vi "CreateObstacleMap.vi"(8 "Base Map":dbl[][](array[numeric]), 11 "Obstacles":T1) -> (3 "Obstacle Map":dbl[][](array[numeric]))   [LabVIEW 2011]
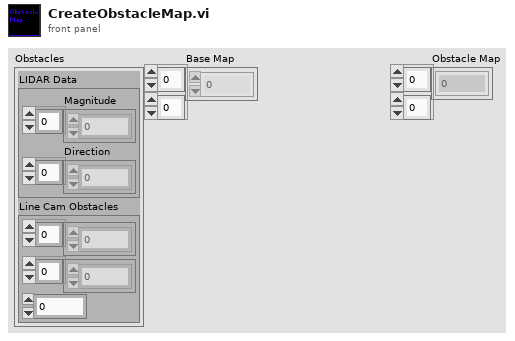
[diagram p1: front panel]
types:
  T1 = cluster{"LIDAR Data":cluster{"Magnitude":dbl[], "Direction":dbl[]}, "Line Cam Obstacles":cluster{dbl[], dbl[], i32}}
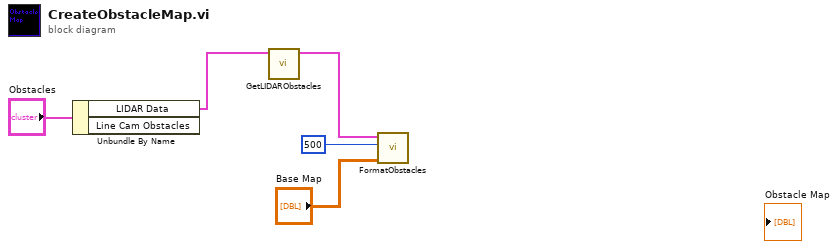
[diagram p0: block diagram]
diagram:
  n1 = Unbundle By Name("Obstacles") -> ("LIDAR Data"=w4:cluster{"Magnitude":dbl[], "Direction":dbl[]})  [unwired: 1 out]
  n2 = call "GetLIDARObstacles.vi"("LIDAR data"=w4) -> ("LIDAR obstacles"=w3:cluster{dbl[], dbl[], i32})  [unwired: 10 in]
  n3 = call "FormatObstacles.vi"("Map In"="Base Map", "Intensity of object"=500, "Obstacles"=w3) -> ()  [unwired: 7 in, 1 out]
